vi "CrossCorrelation (single).vi"(8 "error in (no error)":errorcluster, 10 "XY-data b":cluster{"X-array":dbl[], "Y-array":dbl[]} {"Y-array" format="%.2p"; "X-array" format="%.2p"}, 11 "XY-data a":cluster{"X-array":dbl[], "Y-array":dbl[]} {"Y-array" format="%.2p"; "X-array" format="%.2p"}) -> (0 "error out":errorcluster, 2 "R_ab":cluster{"X-array":dbl[], "Y-array":dbl[]} {"Y-array" format="%.2p"; "X-array" format="%.2p"}, 3 "XY-data out":cluster{"X-array":dbl[], "Y-array":dbl[]} {"Y-array" format="%.2p"; "X-array" format="%.2p"})   [LabVIEW 2019, in "xy_utilities.lvlib"]
doc: "Compute the cross correlation <b>R_ab</b> of <b>XY-data a</b> and <b>XY-data b</b>."
uses:
  xy_utilities.lvlib
  <vilib>/Analysis/2dsp.llb/1D Cross Correlation (DBL).vi
  <vilib>/Analysis/NI_AALPro.lvlib
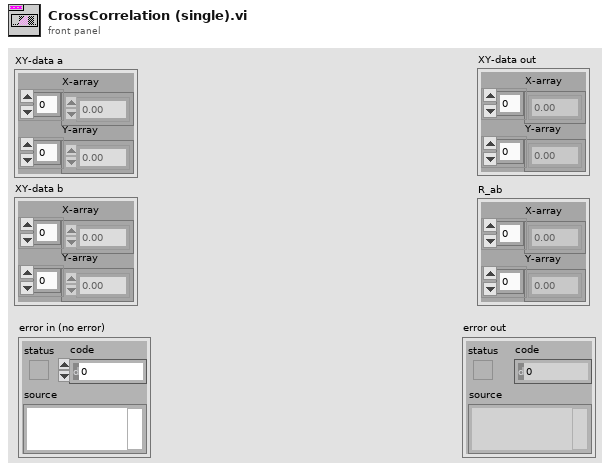
[diagram p1: front panel]
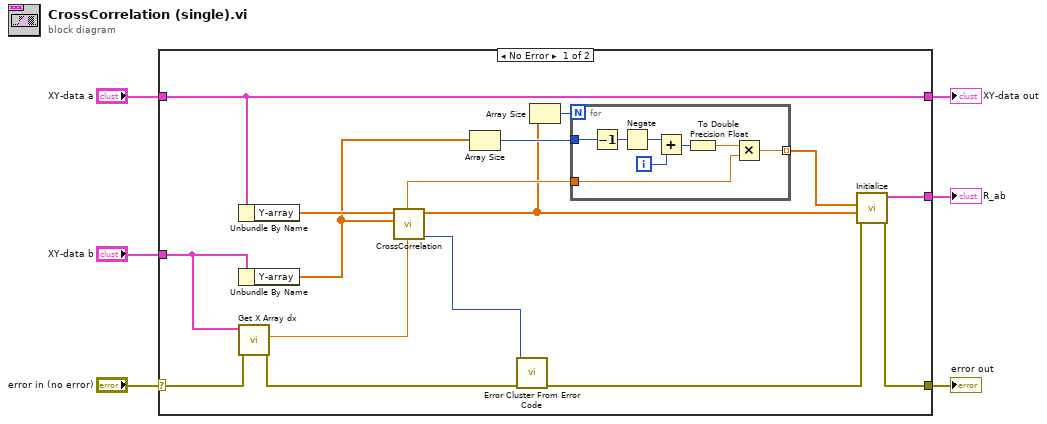
[diagram p0: block diagram]
diagram:
  n1 = case shown="No Error" "error in (no error)" {
    selector: "error in (no error)" -> [w16 w31]
    tunnel: [w13 w31] -> w5
    tunnel: "XY-data a" -> [w12 w30]
    tunnel: [w12 w30] -> w3
    tunnel: "XY-data b" -> [w17 _]
    tunnel: [w11 _] -> w1
    frame No Error {
      n2 = Unbundle By Name(w12) -> ("Y-array"=w20:dbl[])
      n3 = Unbundle By Name(w17) -> ("Y-array"=w7:dbl[])
      n4 = call "Get X Array dx.vi"("error in (no error)"=w16, "XY-data"=w17) -> ("error out"=w9:errorcluster, "dX"=w19:dbl)  [unwired: 6 in, 2 out]
      n5 = call-poly <vilib>:"CrossCorrelation.vi"("Y"=w7, "X"=w20) -> ("error"=w10:i32, "Rxy"=w14:dbl[])  [unwired: 8 in]
      n6 = Array Size(array=w7) -> (size(s)=w18:i32)
      n7 = call <vilib>:"Error Cluster From Error Code.vi"("error in (no error)"=w9, "error code (0)"=w10) -> ("error out"=w8:errorcluster)  [unwired: 7 in]
      n8 = Array Size(array=w14) -> (size(s)=w21:i32)
      n9 = for {
        N: w21 -> [_]
        tunnel: w18 -> [w29]
        tunnel: [w25] -> w15 mode=indexing
        tunnel: w19 -> [w23]
        i -> [w27]
        n10 = Decrement(x=w29) -> (x-1=w28:i32)
        n11 = Negate(x=w28) -> (-x=w24:i32)
        n12 = Add(x=w24, y=w27) -> (x+y=w26:i32)
        n13 = To Double Precision Float(number=w26) -> (double precision float=w22:dbl)
        n14 = Multiply(x=w22, y=w23) -> (x*y=w25:dbl)
      }
      n15 = call "Initialize.vi"("error in (no error)"=w8, "Y-array"=w14, "X-array"=w15) -> ("error out"=w13:errorcluster, "XY-data out"=w11:cluster{"X-array":dbl[], "Y-array":dbl[]})  [unwired: 7 in]
    }
    frame Error {
    }
  }
  "error out" <- w5
  "XY-data out" <- w3
  "R_ab" <- w1
